vi "Configure Marker Function.vi"(7 "State (T: On)":bool=TRUE, 8 "error in (no error)":errorcluster, 9 "Marker Function (0: Flatness)":u16(ring) items=["Flatness", "RF Filter Statistics", "Statistics"], 10 "Channel (1)":i32=1, 11 "VISA resource name":refnum<visa-resource-name>) -> (0 "error out":errorcluster, 3 "VISA resource name out":refnum<visa-resource-name>)   [LabVIEW 2022 SP3, in "Agilent ENA Series.lvlib"]
doc: "Configures the marker function.\n\nNotes:\n(1) This VI is available only for E5061A/B and E5062A."
uses:
  <instrlib>/Agilent ENA Series/Agilent ENA Series.lvlib
panel:
  # "On\n\nOff"
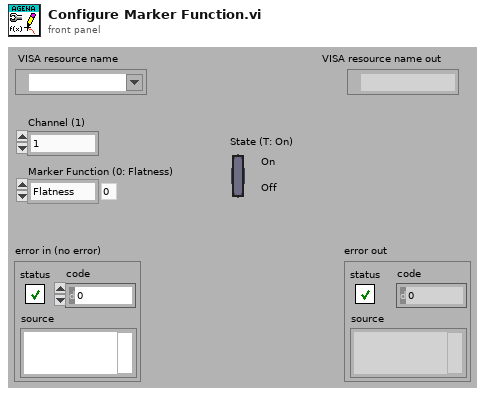
[diagram p1: front panel]
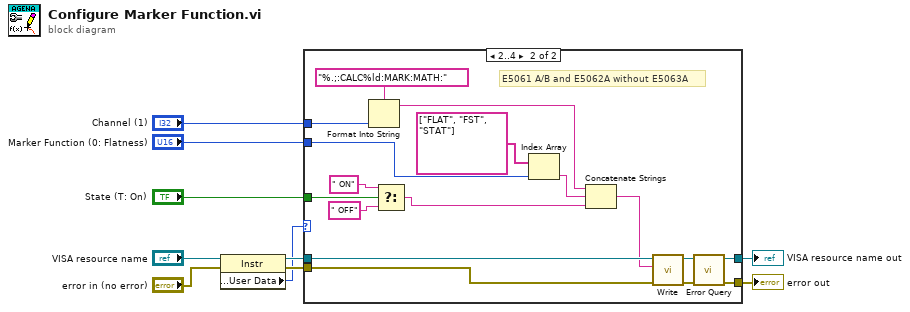
[diagram p0: block diagram]
diagram:
  n1 = property class="Instr"(reference="VISA resource name", error in="error in (no error)") -> (reference out=w10:refnum<visa-resource-name>, error out=w9:errorcluster, "General Settings:User Data"=w1:u32)
  n2 = case shown="2..4" w1 {
    tunnel: w10 -> [w12 w29]
    tunnel: w9 -> [w11 w28]
    tunnel: "Channel (1)" -> [_ w26]
    tunnel: "Marker Function (0: Flatness)" -> [_ w25]
    tunnel: "State (T: On)" -> [_ w24]
    tunnel: [w12 w21] -> w3
    tunnel: [w11 w20] -> w2
    frame 0, Default {
    }
    frame 2..4 {
      # "E5061 A/B and E5062A without E5063A"
      n3 = Format Into String(format string="%.;:CALC%ld:MARK:MATH:", w26) -> (resulting string=w16:string)  [unwired: 2 in, 1 out]
      n4 = Select(t=" ON", s=w24, f=" OFF") -> (s? t:f=w13:string)
      n5 = Index Array(array=string[] ["FLAT", "FST", "STAT"], index=w25) -> (element=w17:string)
      n6 = Concatenate Strings(w16, w17, w13) -> (w27:string)
      n7 = call <instrlib>:"Write.vi"("error in (no error)"=w28, "String ()"=w27, "VISA resource name"=w29) -> ("error out"=w22:errorcluster, "VISA resource name out"=w23:refnum<visa-resource-name>)  [unwired: 6 in, 1 out]
      n8 = call <instrlib>:"Error Query.vi"("error in (no error)"=w22, "VISA resource name"=w23) -> ("error out"=w20:errorcluster, "VISA resource name out"=w21:refnum<visa-resource-name>)  [unwired: 6 in, 2 out]
    }
  }
  "VISA resource name out" <- w3
  "error out" <- w2
